vi "Read configuration.vi"(7 "force loading?":bool=TRUE, 8 "error in (no error)":errorcluster, 11 "Tomo in":refnum<class "Tomo.lvclass">) -> (0 "error out":errorcluster, 3 "Tomo out":refnum<class "Tomo.lvclass">)   [LabVIEW 2012, in "Tomo.lvclass"]
doc: "Reads the XML-based configuration file and populates the configuration cluster accordingly. Configuration file name is <component ID>.xml."
uses:
  Tomo.lvclass
  <vilib>/Distrio/Murmex/Murmex/Murmex.lvclass
  Tomo.lvclass/Tomo.ctl
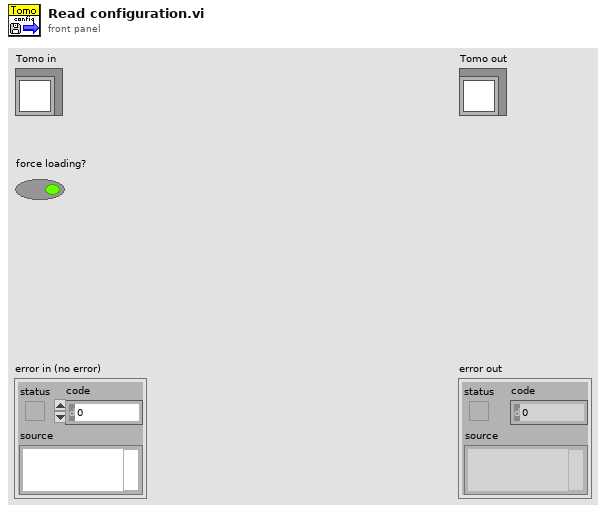
[diagram p1: front panel]
types:
  T1 = typedef "Tomo.lvclass/configuration cluster.ctl" = cluster{"stack component":string, "camera component":string, "stages component":string, "mapping file folder":path, "default stages speed":dbl[unit], "stack overhead time":dbl[unit], "autofocus component":string, "imaging component":string, "AOTF component":string}
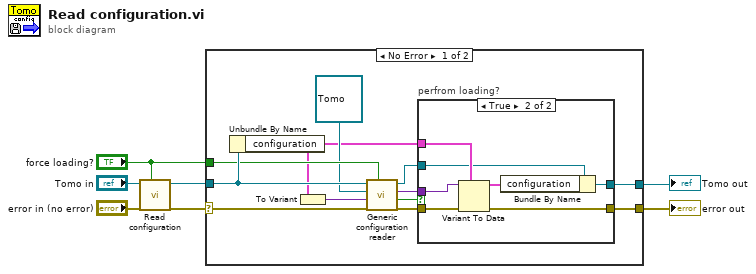
[diagram p0: block diagram]
diagram:
  n1 = call-parent "Read configuration.vi"("force loading?"="force loading?", "error in (no error)"="error in (no error)", "Murmex in"="Tomo in") -> ("error out"=w5:errorcluster, "Murmex out"=w4:refnum<class "Tomo.lvclass">)  [unwired: 7 in]
  n2 = case shown="No Error" w5 {
    selector: w5 -> [w19 w30]
    tunnel: w4 -> [w18 w29]
    tunnel: "force loading?" -> [w17 _]
    tunnel: [w9 w29] -> w2
    tunnel: [w8 w30] -> w1
    frame No Error {
      n3 = Unbundle By Name(w18) -> ("configuration"=w11:T1)
      n4 = To Variant(anything=w11) -> (Variant=w16:variant)
      n5 = call <vilib>:"Generic configuration reader.vi"("force loading?"=w17, "error in (no error)"=w19, "configuration cluster variant"=w16, "inheritance level"=refnum<class "Tomo.lvclass"> refnum ("Tomo.lvclass"), "Murmex in"=w18) -> ("error out"=w13:errorcluster, "loaded?"=w14:bool, "configuration data (variant)"=w12:variant, "Murmex out"=w10:refnum<class "Tomo.lvclass">)  [unwired: 3 in]
      n6 = case "perfrom loading?" shown="True" w14 {
        tunnel: w13 -> [w21 w28]
        tunnel: w12 -> [_ w27]
        tunnel: w11 -> [_ w26]
        tunnel: w10 -> [w20 w25]
        tunnel: [w20 w23] -> w9
        tunnel: [w21 w22] -> w8
        frame False {
        }
        frame True {
          n7 = Variant To Data(error in=w28, type=w26, Variant=w27) -> (data=w24:T1, error out=w22:errorcluster)
          n8 = Bundle By Name(cluster=w25, "configuration"=w24) -> (w23:refnum<class "Tomo.lvclass">)
        }
      }
    }
    frame Error {
    }
  }
  "error out" <- w1
  "Tomo out" <- w2
